vi "FPGAcode5_Debug.vi"(6 "Limits":T1={"High Charge Limit"=4.54747350780585e-13, "Low Charge Limit"=0.0, "High Velocity Limit"=262143.0, "Low Velocity Limit"=0.0, "High Mass Limit"=7.27595761248936e-12, "Low Mass Limit"=0.0, "High Voltage"=2200000.0}, 7 "Speed Bracket":i32, 8 "Thresholds in":i32[](array[numeric])=[0, 0, 0, 0, 0, 0, 0, 0, 0, 0, 0], 9 "Clock Speed (Hz)":i32=40000000, 10 "Calibrate":bool=TRUE, 11 "Detector Waveform In":sgl[][](array[numeric])) -> (0 "Thresholds out":i32[](array[numeric]), 1 "V-M-C Estimate":sgl[](array[numeric]), 3 "PSU Response":bool[](array[boolean]), 5 "Max Stop Point":cluster{"Max Stop":u8, "Index":i32})   [LabVIEW 2015]
uses:
  FPGA3/Detector_Cluster.ctl
  FPGA3/Correlations.ctl
  FPGA3/Limits_In.ctl
panel:
  in  "User Trigger?":bool
  in  "User Trigger Distance":fxp<+/-,34,18> format="%.3g"
  out "User Trigger":bool
  in  "Charge Error Factor":fxp<+,32,0>=0.30000000004656613 format="%_2g"
  in  "Threshold Factor":fxp<+/-,32,16>=1.1999664306640625 format="%.2g"
  out "DCS 2":bool
  out "DCS 1":bool
  in  "Armed":bool
  out "Plates":bool
  in  "One Shot":bool
  # "These factors above are in the front\npanel so it is possible to experiment\nwith different configurations of the\nFPGA on the fly."
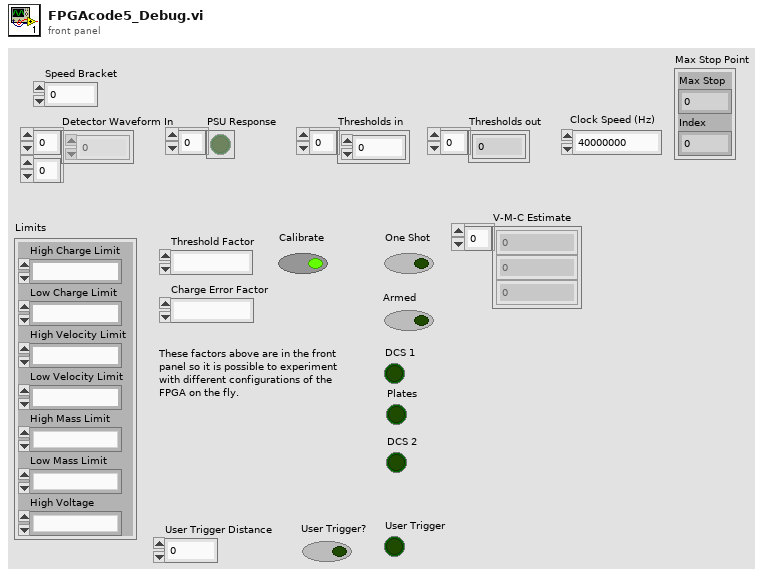
[diagram p1: front panel]
types:
  T1 = typedef "Limits_In.ctl" = cluster{"High Charge Limit":fxp<+,32,-41>, "Low Charge Limit":fxp<+,32,-41>, "High Velocity Limit":fxp<+,18,18>, "Low Velocity Limit":fxp<+,18,18>, "High Mass Limit":fxp<+/-,33,-36>, "Low Mass Limit":fxp<+/-,33,-36>, "High Voltage":fxp<+,32,22>}
  T2 = typedef "Detector_Cluster.ctl" = cluster{"Det 1":i32, "Det 2":i32}
  T3 = cluster{"Filter 1":T2, "Filter 2":T2, "Filter 3":T2, "Filter 4":T2}
  T4 = cluster{"Distance to PSU":fxp<+/-,32,5>, "Distance to end of PSU":fxp<+/-,32,5>, "Distance to DCS 2":fxp<+/-,32,5>, "Distance to DCS 1":fxp<+/-,32,5>, "Distance to front of LEIL Chamber":fxp<+/-,32,5>}
  T5 = cluster{"Detector Max Speed Count":i32, "Detector Min Speed Count":i32, "Gap Max Speed Count":i32, "Gap Min Speed Count":i32}
  T6 = cluster{"Distance to PSU":fxp<+/-,64,37>, "Distance to end of PSU":fxp<+/-,64,37>, "Distance to DCS 2":fxp<+/-,64,37>, "Distance to DCS 1":fxp<+/-,64,37>, "Distance to front of LEIL Chamber":fxp<+/-,64,37>}
  T7 = cluster{"Filter 1":T2, "Filter 2":T2, "Filter 3":T2, "Filter 4":T2}[]
  T8 = cluster{"First Detector Count":i32, "Detector Gap Count":i32, "Second Detector Count":i32, "Second Detector Final Count":i32}
  T9 = typedef "Correlations.ctl" = cluster{"First Correlation":i32, "Latest Correlation":i32}
  T10 = cluster{cluster{i16, i16}, cluster{"Det 1":i16, "Det 2":i16}, cluster{"Det 1":i16, "Det 2":i16}, cluster{"Det 1":i16, "Det 2":i16}}
  T11 = cluster{cluster{"Det 1":i16, "Det 2":i16}, cluster{"Det 1":i16, "Det 2":i16}, cluster{"Det 1":i16, "Det 2":i16}, cluster{"Det 1":i16, "Det 2":i16}}
  T12 = cluster{"Distance to PSU":fxp<+/-,64,69>, "Distance to end of PSU":fxp<+/-,64,69>, "Distance to DCS 2":fxp<+/-,64,69>, "Distance to DCS 1":fxp<+/-,64,69>, "Distance to front of LEIL Chamber":fxp<+/-,64,69>}
  T13 = cluster{"Distance to PSU":i32, "Distance to end of PSU":i32, "Distance to DCS 2":i32, "Distance to DCS 1":i32, "Distance to front of LEIL Chamber":i32}
  T14 = cluster{fxp<+,64,32>, fxp<+/-,64,-31>, "High Charge Limit":fxp<+,32,-41>}
  T15 = cluster{dbl, fxp<+/-,64,-31>, "High Charge Limit":fxp<+,32,-41>}
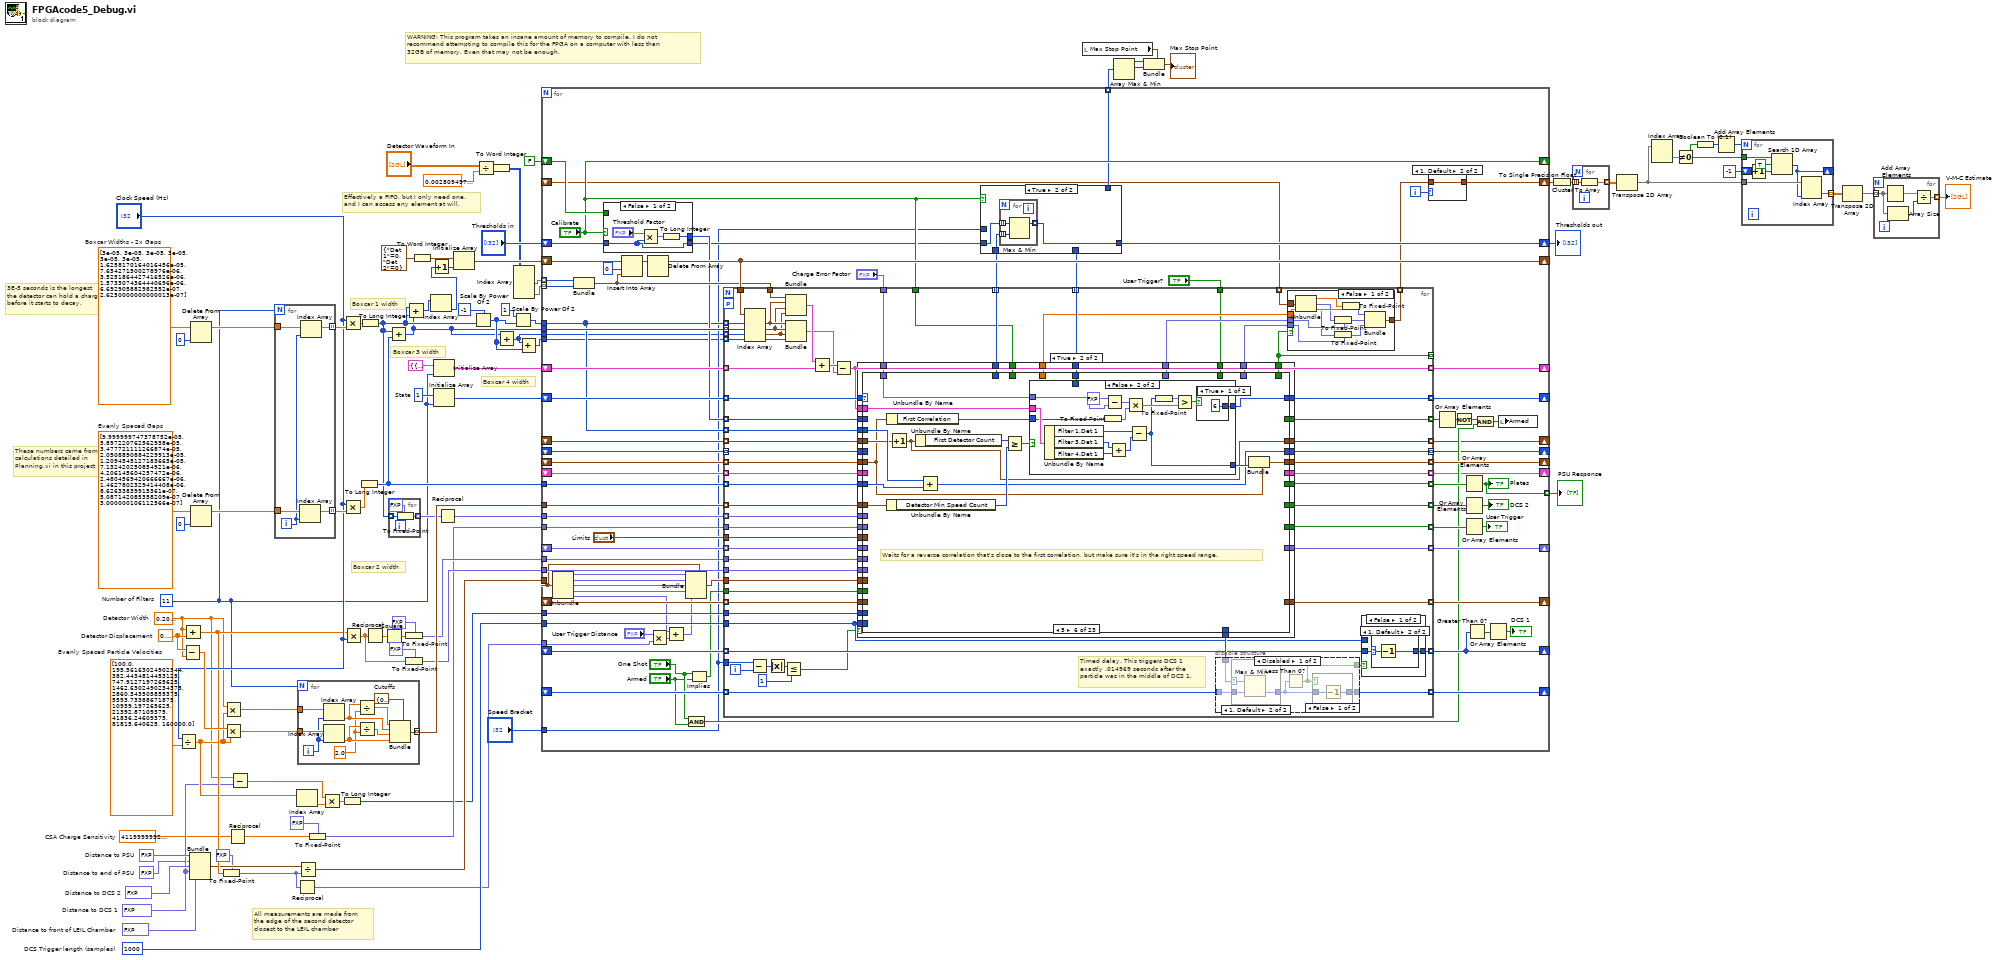
[diagram p0: block diagram]
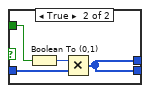
[diagram p3: hidden frame]
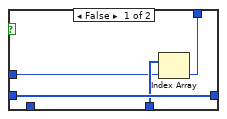
[diagram p4: hidden frame]
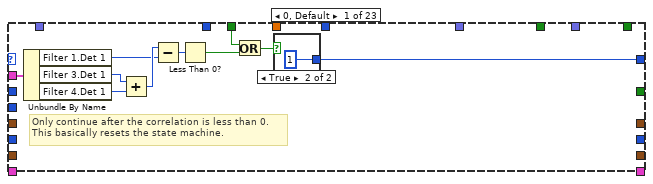
[diagram p6: hidden frame]
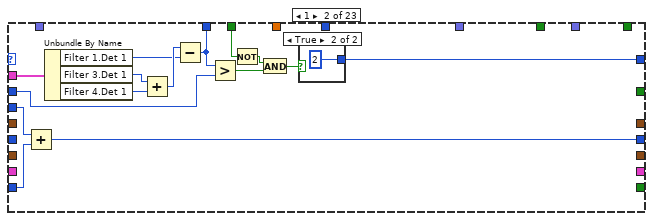
[diagram p8: hidden frame]
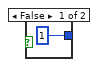
[diagram p9: hidden frame]
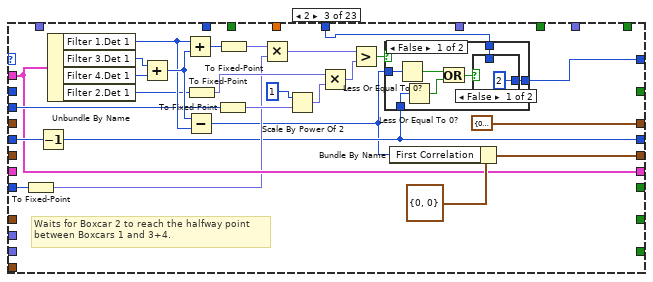
[diagram p10: hidden frame]
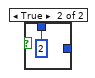
[diagram p11: hidden frame]
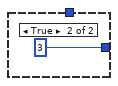
[diagram p12: hidden frame]
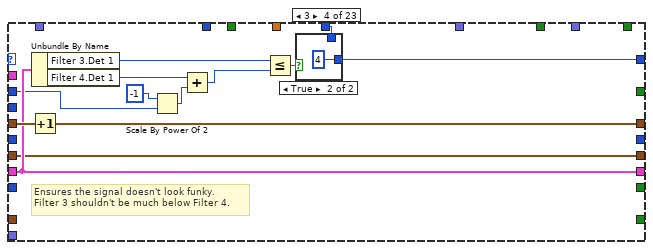
[diagram p13: hidden frame]
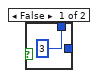
[diagram p14: hidden frame]
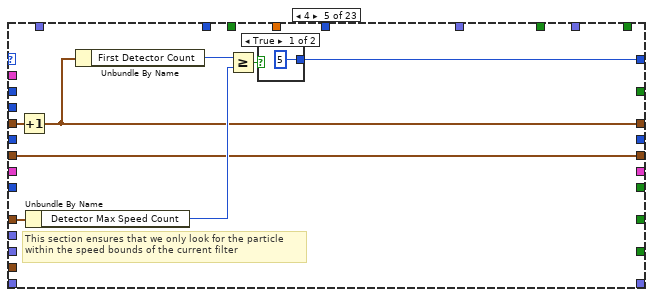
[diagram p15: hidden frame]
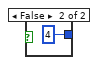
[diagram p16: hidden frame]
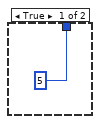
[diagram p17: hidden frame]
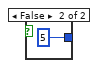
[diagram p18: hidden frame]
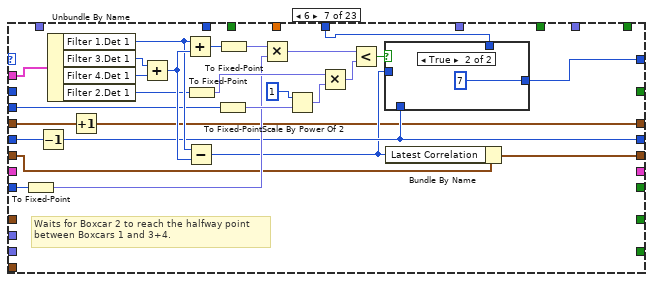
[diagram p19: hidden frame]
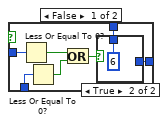
[diagram p20: hidden frame]
diagram:
  w30 = dbl[] [3e-05, 3e-05, 3e-05, 3e-05, 3e-05, 3e-05, 1.6258170164016456e-05, 7.654271500278976e-06, 3.5251864427416526e-06, 1.5733074364440696e-06, 6.692905882982552e-07, 2.6250000000000013e-07]  # Boxcar Widths - 2x Gaps
  w43 = fxp<+/-,32,5> 4.297679997980595  # Distance to front of LEIL Chamber
  w49 = u16 1000  # DCS Trigger length (samples)
  w54 = fxp<+/-,32,5> -1.3589000031352043  # Distance to DCS 1
  w57 = fxp<+/-,32,5> 2.6162000000476837  # Distance to DCS 2
  w46 = fxp<+/-,32,5> 2.7999999970197678  # Distance to end of PSU
  w58 = fxp<+/-,32,5> 0.10000000149011612  # Distance to PSU
  w42 = sgl 4120000000000000.0  # CSA Charge Sensitivity
  w89 = u8 1  # State
  w55 = sgl 0.6  # Detector Displacement
  w93 = sgl[] [0.0001, 5.8972208e-05, 3.477721e-05, 2.050889e-05, 1.2094545e-05, 7.1324203e-06, 4.2061456e-06, 2.480457e-06, 1.4627802e-06, 8.6263384e-07, 5.087142e-07, 3e-07]  # Evenly Spaced Gaps
  w74 = sgl[] [100.0, 195.56163, 382.44348, 747.9127, 1462.6302, 2860.3435, 5593.734, 10939.197, 21392.871, 41836.246, 81815.64, 160000.0]  # Evenly Spaced Particle Velocities
  w50 = sgl 0.21  # Detector Width
  w47 = 11  # Number of Filters
  # "WARNING: This program takes an insane amount of memory to compile. I do not\nrecommend attempting to compile this for the FPGA on a computer with less than\n32GB of memory. Even that may not be enough."
  # "Boxcar 3 width"
  # "Boxcar 4 width"
  # "All measurements are made from\nthe edge of the second detector\nclosest to the LEIL chamber"
  # "Effectively a FIFO, but I only need one,\nand I can access any element at will."
  # "Boxcar 2 width"
  # "Boxcar 1 width"
  # "3E-5 seconds is the longest\nthe detector can hold a charge\nbefore it starts to decay."
  # "These numbers came from\ncalculations detailed in\nPlanning.vi in this project"
  n1 = Divide(x="Clock Speed (Hz)", y=w74) -> (x/y=w56:sgl[])
  n2 = Subtract(x=w55, y=w50) -> (x-y=w73:sgl)
  n3 = Add(x=w50, y=w55) -> (x+y=w61:sgl)
  n4 = Bundle("Distance to PSU"=w58, "Distance to end of PSU"=w46, "Distance to DCS 2"=w57, "Distance to DCS 1"=w54, "Distance to front of LEIL Chamber"=w43) -> (w60:T4)  [unwired: 1 in]
  n5 = Delete From Array(array=w30, index=0) -> (array with subset deleted=w82:dbl[])  [unwired: 1 in, 1 out]
  n6 = Delete From Array(array=w93, index=0) -> (array with subset deleted=w84:sgl[])  [unwired: 1 in, 1 out]
  n7 = To Fixed-Point(fixed-point type=fxp<+/-,32,1> 0.0, number=w61) -> (fixed-point=w45:fxp<+/-,32,1>)
  n8 = Multiply(x=w50, y=w56) -> (x*y=w91:sgl[])
  n9 = Multiply(x=w73, y=w56) -> (x*y=w92:sgl[])
  n10 = Reciprocal(x=w42) -> (1/x=w63:sgl)
  n11 = Subtract(x=w50, y=w54) -> (x-y=w52:sgl)
  n12 = for {
    N: w47 -> [_]
    tunnel: w84 -> [w101]
    tunnel: [w98] -> w83 mode=indexing
    tunnel: w82 -> [w100]
    tunnel: [w99] -> w81 mode=indexing
    i -> [w97]
    n13 = Index Array(array=w101, index=w97) -> (element=w98:sgl)
    n14 = Index Array(array=w100, index=w97) -> (element=w99:dbl)
  }
  n15 = Index Array(array=w56) -> (element=w53:sgl)  [unwired: 1 in]
  n16 = Reciprocal(x=w45) -> (1/x=w44:fxp<+/-,34,33>)
  n17 = for {
    N: w47 -> [_]
    tunnel: w92 -> [w111]
    tunnel: w91 -> [w110]
    tunnel: [w109] -> w86 mode=indexing
    i -> [w108]
    w102 = sgl 2.0 ("y")
    w107 = T5 {"Detector Max Speed Count"=0, "Detector Min Speed Count"=0, "Gap Max Speed Count"=0, "Gap Min Speed Count"=0}  # Cutoffs
    n18 = Index Array(array=w110, index=w108) -> (element=w106:sgl)
    n19 = Index Array(array=w111, index=w108) -> (element=w103:sgl)
    n20 = Divide(x=w106, y=w102) -> (x/y=w105:sgl)
    n21 = Divide(x=w103, y=w102) -> (x/y=w104:sgl)
    n22 = Bundle(cluster=w107, "Detector Max Speed Count"=w105, "Detector Min Speed Count"=w106, "Gap Max Speed Count"=w104, "Gap Min Speed Count"=w103) -> (w109:T5)
  }
  n23 = Divide(x=w60, y=w45) -> (x/y=w59:T6)
  n24 = To Fixed-Point(fixed-point type=fxp<+,32,-49> 0.0, number=w63) -> (fixed-point=w62:fxp<+,32,-49>)
  n25 = Multiply(x=w52, y=w53) -> (x*y=w51:sgl)
  n26 = To Long Integer(number=w51) -> (32bit integer=w48:i32)
  n27 = Multiply(x="Clock Speed (Hz)", y=w81) -> (x*y=w85:dbl[])
  n28 = Multiply(x="Clock Speed (Hz)", y=w83) -> (x*y=w90:sgl[])
  n29 = Multiply(x=w61, y="Clock Speed (Hz)") -> (x*y=w66:sgl)
  n30 = To Long Integer(number=w90) -> (32bit integer=w80:i32[])
  n31 = To Long Integer(number=w85) -> (32bit integer=w6:i32[])
  n32 = Reciprocal(x=w66) -> (1/x=w70:sgl)
  n33 = Square(x=w70) -> (x^2=w69:sgl)
  n34 = Add(x=w6, y=w80) -> (x+y=w2:i32[])
  n35 = for {
    tunnel: w6 -> [w114] mode=indexing
    tunnel: [w113] -> w76 mode=indexing
    n36 = To Fixed-Point(fixed-point type=fxp<+/-,32,32> 0.0, number=w114) -> (fixed-point=w113:fxp<+/-,32,32>)
  }
  n37 = To Fixed-Point(fixed-point type=fxp<+/-,32,-42> 0.0, number=w69) -> (fixed-point=w72:fxp<+/-,32,-42>)
  n38 = To Fixed-Point(fixed-point type=fxp<+,32,28> 0.0, number=w66) -> (fixed-point=w64:fxp<+,32,28>)
  n39 = Add(x=w6, y=w2) -> (x+y=w38:i32[])
  n40 = To Word Integer(number=T2 {"Det 1"=0, "Det 2"=0} ("Detectors")) -> (16bit integer=w79:cluster{"Det 1":i16, "Det 2":i16})
  n41 = Index Array(array=w38) -> (element=w37:i32)  [unwired: 1 in]
  n42 = Increment(x=w37) -> (x+1=w36:i32)
  n43 = Initialize Array(T3 {"Filter 1"={"Det 1"=0, "Det 2"=0}, "Filter 2"={"Det 1"=0, "Det 2"=0}, "Filter 3"={"Det 1"=0, "Det 2"=0}, "Filter 4"={"Det 1"=0, "Det 2"=0}} ("cluster"), w47) -> (w87:T7)
  n44 = Initialize Array(w89, w47) -> (w88:u8[])
  n45 = Reciprocal(x=w76) -> (1/x=w75:fxp<+/-,34,2>[])
  n46 = Initialize Array(w79, w36) -> (w96:cluster{"Det 1":i16, "Det 2":i16}[])
  n47 = Scale By Power Of 2(n=i16 -1, x=w6) -> (x*2^n=w4:i32[])
  n48 = Divide(x="Detector Waveform In", y=sgl 0.0028094975 ("min value")) -> (x/y=w41:sgl[][])
  n49 = To Word Integer(number=w41) -> (16bit integer=w31:i16[][])
  n50 = Add(x=w2, y=w4) -> (x+y=w5:i32[])
  n51 = Scale By Power Of 2(n=i16 1, x=w4) -> (x*2^n=w9:i32[])
  n52 = Index Array(array=w31) -> (element #1=w33:i16[], element #2=w32:i16[])  [unwired: 4 in]
  n53 = Add(x=w5, y=w4) -> (x+y=w3:i32[])
  n54 = for {
    shift-right: [w196] -> _
    shift-left: w96 -> [w197]
    shift-right: [w121] -> _
    shift-left: w87 -> [w193]
    shift-right: [w123] -> _
    shift-left: w88 -> [w195]
    shift-right: [w122] -> _
    shift-left: _ -> [w194]
    tunnel: w86 -> [w192]
    shift-right: [w191] -> _
    shift-left: _ -> [w190]
    tunnel: w9 -> [w120]
    tunnel: w2 -> [w189]
    tunnel: w80 -> [w188]
    tunnel: w75 -> [w187]
    shift-right: [w186] -> _
    shift-left: _ -> [w185]
    tunnel: w72 -> [w184]
    tunnel: w62 -> [w183]
    tunnel: w64 -> [w182]
    tunnel: w59 -> [w169]
    shift-right: [w181] -> _
    shift-left: _ -> [w180]
    shift-right: [w179] -> w39
    shift-left: "Thresholds in" -> [w178]
    shift-right: ["Calibrate"] -> _
    shift-left: FALSE ("Calibrate") -> [w177]
    tunnel: w49 -> [w176]
    tunnel: w48 -> [w175]
    shift-right: [w173] -> _
    shift-left: _ -> [w174]
    shift-right: [w172] -> _
    shift-left: _ -> [w171]
    tunnel: w44 -> [w170]
    tunnel: [w136] -> w29 mode=indexing
    shift-right: [w135] -> _
    shift-left: _ -> [w134]
    tunnel: w33 -> [w133] mode=indexing
    tunnel: w32 -> [w132] mode=indexing
    tunnel: [w128] -> w28 mode=indexing
    tunnel: "Speed Bracket" -> [w117]
    shift-right: [w125] -> w18
    shift-left: _ -> [w127]
    shift-right: [w119] -> _
    shift-left: _ -> [w118]
    tunnel: w3 -> [w116]
    tunnel: w5 -> [w115]
    i -> [w126]
    n55 = Unbundle(w169) -> ("Distance to PSU"=w158:fxp<+/-,64,37>, "Distance to end of PSU"=w157:fxp<+/-,64,37>, "Distance to DCS 2"=w156:fxp<+/-,64,37>, "Distance to DCS 1"=w153:fxp<+/-,64,37>, "Distance to front of LEIL Chamber"=w152:fxp<+/-,64,37>)
    n56 = Bundle(w133, w132) -> (w137:cluster{i16, i16})  [unwired: 1 in]
    n57 = case shown="False" "Calibrate" {
      tunnel: w178 -> [w200 w206]
      tunnel: [w200 w203] -> w129
      tunnel: w177 -> [_ w205]
      tunnel: [w199 w203] -> w130
      frame False {
        n58 = Multiply(x="Threshold Factor", y=w200) -> (x*y=w201:fxp<+/-,64,48>[])
        n59 = To Long Integer(number=w201) -> (32bit integer=w199:i32[])
      }
      frame True {
        n60 = Boolean To (0,1)(Boolean=w205) -> (0, 1=w204:i16)
        n61 = Multiply(x=w204, y=w206) -> (x*y=w203:i32[])
      }
    }
    n62 = Insert Into Array(array=w197, index=0, new element=w137) -> (w168:cluster{"Det 1":i16, "Det 2":i16}[])
    n63 = Delete From Array(array=w168) -> (array with subset deleted=w196:cluster{"Det 1":i16, "Det 2":i16}[])  [unwired: 2 in, 1 out]
    n64 = Multiply(x="User Trigger Distance", y=w170) -> (x*y=w154:fxp<+/-,64,49>)
    n65 = Add(x=w152, y=w154) -> (x+y=w151:fxp<+/-,64,50>)
    n66 = Bundle(cluster=w169, "Distance to PSU"=w158, "Distance to end of PSU"=w157, "Distance to DCS 2"=w156, "Distance to DCS 1"=w153, "Distance to front of LEIL Chamber"=w151) -> (w155:T6)
    n67 = And(x="One Shot", y="Armed") -> (x .and. y?=w142:bool)
    n68 = Implies(1:"Armed", 2:"One Shot") -> (0:w162:bool)
    n69 = for {
      tunnel: w196 -> [w285]
      tunnel: [w271] -> w121 mode=indexing
      tunnel: w195 -> [w284] mode=indexing
      tunnel: [w283] -> w123 mode=indexing
      tunnel: w130 -> [w220] mode=indexing
      tunnel: [w282] -> w122 mode=indexing
      tunnel: w194 -> [w281] mode=indexing
      tunnel: w193 -> [w275] mode=indexing
      tunnel: w137 -> [w280]
      tunnel: w192 -> [w270] mode=indexing
      tunnel: [w269] -> w191 mode=indexing
      tunnel: w190 -> [w268] mode=indexing
      tunnel: w120 -> [w267] mode=indexing
      tunnel: w189 -> [w218] mode=indexing
      tunnel: w115 -> [w266] mode=indexing
      tunnel: w116 -> [w265] mode=indexing
      tunnel: w120 -> [w226] mode=indexing
      tunnel: w188 -> [w225] mode=indexing
      tunnel: "Charge Error Factor" -> [w264]
      tunnel: [w263] -> w164 mode=indexing
      tunnel: w187 -> [w262] mode=indexing
      tunnel: "Limits" -> [w261]
      tunnel: [w260] -> w186 mode=indexing
      tunnel: w185 -> [w259] mode=indexing
      tunnel: w184 -> [w258]
      tunnel: w183 -> [w257]
      tunnel: w182 -> [w256]
      tunnel: w155 -> [w255]
      tunnel: [w254] -> w181 mode=indexing
      tunnel: w180 -> [w253] mode=indexing
      tunnel: [w252] -> w163 mode=indexing
      tunnel: w162 -> [w251]
      tunnel: w176 -> [w248]
      tunnel: w175 -> [w250]
      tunnel: [w247] -> w173 mode=indexing
      tunnel: w174 -> [w246] mode=indexing
      tunnel: [w244] -> w172 mode=indexing
      tunnel: w171 -> [w243] mode=indexing
      tunnel: [w242] -> w150 mode=indexing
      tunnel: [w241] -> w149 mode=indexing
      tunnel: [w240] -> w148 mode=indexing
      tunnel: [w239] -> w145 mode=indexing
      tunnel: "User Trigger?" -> [w235]
      tunnel: w134 -> [w233] mode=indexing
      tunnel: [w232] -> w135 mode=indexing
      tunnel: "Calibrate" -> [w231]
      tunnel: [w224] -> w124 mode=indexing
      tunnel: w127 -> [w230] mode=indexing
      workers-P: _ -> [_]
      tunnel: w117 -> [w221]
      tunnel: [w223] -> _ mode=indexing
      tunnel: [w219] -> w119 mode=indexing
      tunnel: w118 -> [w217] mode=indexing
      i -> [w222]
      # "Timed delay. This triggers DCS 1\nexactly .014969 seconds after the\nparticle was in the middle of DCS 1."
      n70 = Index Array(array=w285, index #1=w267, index #2=w218, index #3=w266, index #4=w265) -> (element #1=w278:cluster{"Det 1":i16, "Det 2":i16}, element #2=w277:cluster{"Det 1":i16, "Det 2":i16}, element #3=w276:cluster{"Det 1":i16, "Det 2":i16}, element #4=w279:cluster{"Det 1":i16, "Det 2":i16})
      n71 = Subtract(x=w221, y=w222) -> (x-y=w234:i32)
      n72 = Absolute Value(x=w234) -> (abs(x)=w229:i32)
      n73 = Less Or Equal?(x=w229, y=1) -> (x <= y?=w228:bool)
      n74 = Bundle(w280, w278, w277, w276) -> (w274:T10)  [unwired: 1 in]
      n75 = Bundle(w278, w277, w276, w279) -> (w272:T11)  [unwired: 1 in]
      n76 = Add(x=w274, y=w275) -> (x+y=w273:T3)
      n77 = Subtract(x=w273, y=w272) -> (x-y=w271:T3)
      n78 = case shown="True" w228 {
        tunnel: w284 -> [_ w327]
        tunnel: w220 -> [_ w326]
        tunnel: [_ w325] -> w283
        tunnel: [_ w324] -> w282
        tunnel: w281 -> [_ w323]
        tunnel: w217 -> [_ w322]
        tunnel: w271 -> [_ w321]
        tunnel: w270 -> [_ w320]
        tunnel: [_ w319] -> w269
        tunnel: w268 -> [_ w318]
        tunnel: w225 -> [_ w317]
        tunnel: w264 -> [_ w316]
        tunnel: [_ w315] -> w263
        tunnel: w262 -> [_ w314]
        tunnel: w261 -> [_ w313]
        tunnel: [_ w312] -> w260
        tunnel: w259 -> [_ w311]
        tunnel: w258 -> [_ w310]
        tunnel: w257 -> [_ w309]
        tunnel: w256 -> [_ w308]
        tunnel: w255 -> [_ w307]
        tunnel: [_ w306] -> w254
        tunnel: w253 -> [_ w305]
        tunnel: [_ w304] -> w252
        tunnel: w251 -> [_ w303]
        tunnel: w250 -> [_ w302]
        tunnel: [_ w301] -> w249
        tunnel: w248 -> [_ w300]
        tunnel: [_ w299] -> w242
        tunnel: [_ w298] -> w241
        tunnel: [_ w297] -> w240
        tunnel: [_ w296] -> w239
        tunnel: [_ w295] -> w238
        tunnel: [_ w294] -> w237
        tunnel: [_ w293] -> w236
        tunnel: w226 -> [_ w292]
        tunnel: w235 -> [_ w291]
        tunnel: [_ w290] -> w232
        tunnel: w233 -> [_ w289]
        tunnel: [_ w288] -> w223
        tunnel: w231 -> [_ w287]
        tunnel: [_ w286] -> w219
        frame False {
        }
        frame True {
          n79 = case shown="5" w327 {
            tunnel: w326 -> [_ w353 _ w393 _ _ _ _ _ _ _ _ _ _ _ _ _ _ _ _ _ _ _]
            tunnel: [w336 w351 w380 w404 w410 w425 w477 w510 w554 w567 w583 w638 w668 w687 w739 w790 u8 17 ("Det 3") w823 w831 w838 w852 w858 w871] -> w325
            tunnel: w292 -> [_ w341 w371 _ _ w427 w469 _ _ _ w585 _ _ w689 _ _ w814 _ _ _ _ _ _]
            tunnel: [_ _ T8 {"First Detector Count"=0, "Detector Gap Count"=0, "Second Detector Count"=0, "Second Detector Final Count"=0} ("Cutoffs") w398 w407 w417 w452 w508 w550 w572 _ w636 w673 _ w737 _ _ _ _ _ _ _ _] -> w324
            tunnel: w323 -> [_ _ _ w403 w408 w422 w453 w507 w549 w572 w582 w635 w673 w686 w736 _ _ _ _ _ _ _ _]
            tunnel: w322 -> [_ _ w381 _ _ _ w478 w513 _ _ _ w641 _ _ w742 _ _ _ _ _ _ _ _]
            tunnel: w321 -> [w331 w346 w364 _ _ w428 w462 w489 _ _ w586 w633 _ w682 w734 _ _ _ _ _ _ _ _]
            tunnel: w320 -> [_ _ _ _ w414 w433 _ w499 _ w571 w591 w626 w672 w693 w727 _ _ _ _ _ _ _ _]
            tunnel: [_ _ w366 w399 w409 w421 w464 w503 w552 w570 w579 w630 w671 w680 w731 w802 _ _ _ _ _ _ _] -> w319
            tunnel: w318 -> [_ _ _ w399 w409 w419 w454 w511 w553 w573 w592 w639 w674 w694 w740 w803 w821 _ _ _ _ _ _]
            tunnel: w317 -> [_ w340 w372 _ _ w426 w470 _ _ _ w584 _ _ w688 _ _ _ _ _ _ _ _ _]
            tunnel: w316 -> [_ _ _ _ _ w429 _ w491 _ _ w587 w618 _ w690 w721 _ _ _ _ _ _ _ _]
            tunnel: [_ _ w357 w402 _ w430 w456 w493 w555 _ w588 w620 _ w691 w723 w789 _ _ _ _ _ _ _] -> w315
            tunnel: w314 -> [_ _ _ _ _ _ _ _ w560 _ _ _ _ _ _ _ _ _ _ _ _ _ _]
            tunnel: w313 -> [_ _ _ _ _ _ _ _ w563 _ _ _ _ _ _ w804 _ _ _ _ _ _ _]
            tunnel: [_ _ _ _ _ _ _ _ w538 w566 w576 w616 w667 w684 w719 _ _ _ _ _ _ _ _] -> w312
            tunnel: w311 -> [_ _ _ _ _ _ _ _ _ w566 w576 w616 w667 w684 w719 w776 _ _ _ _ _ _ _]
            tunnel: w310 -> [_ _ _ _ _ _ _ _ _ _ _ _ _ _ _ w800 _ _ _ _ _ _ _]
            tunnel: w309 -> [_ _ _ _ _ _ _ _ w547 _ _ _ _ _ _ _ _ _ _ _ _ _ _]
            tunnel: w308 -> [_ _ _ _ _ _ _ _ _ _ _ _ _ _ _ w774 _ _ _ _ _ _ _]
            tunnel: w307 -> [_ _ _ _ _ _ _ _ _ _ _ _ _ _ _ _ w818 _ _ _ _ _ _]
            tunnel: [_ _ _ _ _ _ _ _ _ _ _ _ _ _ _ _ w811 w825 w833 w840 w849 w860 w869] -> w306
            tunnel: w305 -> [_ _ _ _ _ _ _ _ _ _ _ _ _ _ _ _ _ w826 w834 w841 w850 w861 w870]
            tunnel: [_ w345 _ _ _ _ _ _ _ _ _ _ _ _ _ _ _ _ _ _ _ _ _] -> w304
            tunnel: w303 -> [_ _ _ _ _ _ _ _ _ _ _ _ _ _ _ w783 _ _ _ _ _ _ _]
            tunnel: w302 -> [_ _ _ _ _ _ _ _ _ _ _ _ _ _ _ _ w810 _ _ _ _ _ _]
            tunnel: w300 -> [_ _ _ _ _ _ _ _ _ _ _ _ _ _ _ _ _ _ _ _ w847 _ w867]
            tunnel: [_ _ _ _ _ _ _ _ _ _ _ _ _ _ _ _ w808 _ _ _ _ _ _] -> w301
            tunnel: [_ _ _ _ _ _ _ _ _ _ _ _ _ _ _ _ _ _ TRUE _ _ _ _] -> w299
            tunnel: [_ _ _ _ _ _ _ _ _ _ _ _ _ _ _ _ _ _ _ _ TRUE _ _] -> w298
            tunnel: [_ _ _ _ _ _ _ _ _ _ _ _ _ _ _ _ _ _ _ _ _ _ TRUE] -> w297
            tunnel: [_ _ _ _ _ _ _ _ _ _ _ _ _ _ _ w782 _ _ _ _ _ _ _] -> w296
            tunnel: [_ _ _ _ _ _ _ _ _ _ _ _ _ _ _ w773 _ _ _ _ _ _ _] -> w293
            tunnel: [_ _ _ _ _ _ _ _ w538 _ _ _ _ _ _ w776 _ _ _ _ _ _ _] -> w295
            tunnel: [_ _ _ _ _ _ _ _ _ _ _ _ _ _ _ w771 _ _ _ _ _ _ _] -> w294
            tunnel: w291 -> [_ _ _ _ _ _ _ _ _ _ _ _ _ _ _ _ _ _ _ _ w844 _ _]
            tunnel: [_ _ w364 w400 _ _ _ _ _ _ _ _ _ _ _ _ _ _ _ _ _ _ _] -> w290
            tunnel: w289 -> [_ _ _ w400 _ _ _ _ _ _ _ _ _ _ _ _ _ _ _ _ _ _ _]
            tunnel: [_ _ _ _ _ _ _ _ TRUE ("result") _ _ _ _ _ _ TRUE ("result") _ _ _ _ _ _ _] -> w288
            tunnel: w287 -> [w328 w342 _ _ _ _ _ _ _ _ _ _ _ _ _ _ _ _ _ _ _ _ _]
            tunnel: [_ w339 w360 _ _ w418 w458 _ _ _ _ _ _ _ _ _ _ _ _ _ _ _ _] -> w286
            frame 0, Default {
              # "Only continue after the correlation is less than 0.\nThis basically resets the state machine."
              n80 = Unbundle By Name(w331) -> ("Filter 1.Det 1"=w332:i32, "Filter 3.Det 1"=w333:i32, "Filter 4.Det 1"=w334:i32)
              n81 = Add(x=w333, y=w334) -> (x+y=w335:i32)
              n82 = Subtract(x=w335, y=w332) -> (x-y=w330:i32)
              n83 = Less Than 0?(x=w330) -> (x < 0?=w337:bool)
              n84 = Or(x=w328, y=w337) -> (x .or. y?=w329:bool)
              n85 = case shown="True" w329 {
                tunnel: [_ u8 1 ("Det 3")] -> w336
                frame False {
                }
                frame True {
                }
              }
            }
            frame 1 {
              n86 = Add(x=w341, y=w340) -> (x+y=w339:i32)
              n87 = Unbundle By Name(w346) -> ("Filter 1.Det 1"=w347:i32, "Filter 3.Det 1"=w348:i32, "Filter 4.Det 1"=w349:i32)
              n88 = Add(x=w348, y=w349) -> (x+y=w350:i32)
              n89 = Subtract(x=w350, y=w347) -> (x-y=w345:i32)
              n90 = Greater?(x=w345, y=w353) -> (0:w352:bool)
              n91 = Not(x=w342) -> (.not. x?=w343:bool)
              n92 = And(x=w343, y=w352) -> (x .and. y?=w344:bool)
              n93 = case shown="True" w344 {
                tunnel: [u8 1 ("Det 3") u8 2 ("Det 3")] -> w351
                frame False {
                }
                frame True {
                }
              }
            }
            frame 2 {
              # "Waits for Boxcar 2 to reach the halfway point\nbetween Boxcars 1 and 3+4."
              n94 = To Fixed-Point(number=w372) -> (fixed-point=w361:fxp<+/-,32,32>)  [unwired: 1 in]
              n95 = Decrement(x=w381) -> (x-1=w360:i32)
              n96 = Unbundle By Name(w364) -> ("Filter 1.Det 1"=w374:i32, "Filter 3.Det 1"=w378:i32, "Filter 4.Det 1"=w377:i32, "Filter 2.Det 1"=w368:i32)
              n97 = Add(x=w378, y=w377) -> (x+y=w375:i32)
              n98 = Add(x=w374, y=w375) -> (x+y=w379:i32)
              n99 = Subtract(x=w375, y=w374) -> (x-y=w356:i32)
              n100 = To Fixed-Point(number=w368) -> (fixed-point=w363:fxp<+/-,32,32>)  [unwired: 1 in]
              n101 = To Fixed-Point(number=w371) -> (fixed-point=w362:fxp<+/-,32,32>)  [unwired: 1 in]
              n102 = To Fixed-Point(number=w379) -> (fixed-point=w365:fxp<+/-,32,32>)  [unwired: 1 in]
              n103 = Multiply(x=w365, y=w361) -> (x*y=w373:fxp<+/-,64,64>)
              n104 = Scale By Power Of 2(n=i16 1, x=w362) -> (x*2^n=w369:fxp<+/-,32,32>)
              n105 = Multiply(x=w363, y=w369) -> (x*y=w367:fxp<+/-,64,64>)
              n106 = Greater?(x=w373, y=w367) -> (0:w358:bool)
              n107 = case shown="False" w358 {
                tunnel: [w388 u8 3 ("Det 3")] -> w380
                tunnel: w360 -> [w383 _]
                tunnel: [w387 _] -> w357
                tunnel: w356 -> [w382 _]
                frame False {
                  n108 = Less Or Equal To 0?(x=w382) -> (x <= 0?=w385:bool)
                  n109 = Less Or Equal To 0?(x=w383) -> (x <= 0?=w384:bool)
                  n110 = Or(x=w385, y=w384) -> (x .or. y?=w386:bool)
                  n111 = case shown="False" w386 {
                    tunnel: [u8 2 ("Det 3") _] -> w388
                    tunnel: [_ u8 2 ("Det 3")] -> w387
                    frame False {
                    }
                    frame True {
                    }
                  }
                }
                frame True {
                }
              }
              n112 = Bundle By Name(cluster=T9 {"First Correlation"=0, "Latest Correlation"=0}, "First Correlation"=w356) -> (w366:T9)
            }
            frame 3 {
              # "Ensures the signal doesn't look funky.\nFilter 3 shouldn't be much below Filter 4."
              n113 = Increment(x=w403) -> (x+1=w398:T8)
              n114 = Unbundle By Name(w400) -> ("Filter 3.Det 1"=w397:i32, "Filter 4.Det 1"=w396:i32)
              n115 = Scale By Power Of 2(n=i16 -1, x=w393) -> (x*2^n=w392:i32)
              n116 = Add(x=w396, y=w392) -> (x+y=w395:i32)
              n117 = Less Or Equal?(x=w397, y=w395) -> (x <= y?=w401:bool)
              n118 = case shown="True" w401 {
                tunnel: [_ u8 4] -> w404
                tunnel: [u8 3 _] -> w402
                frame False {
                }
                frame True {
                }
              }
            }
            frame 4 {
              # "This section ensures that we only look for the particle\nwithin the speed bounds of the current filter"
              n119 = Increment(x=w408) -> (x+1=w407:T8)
              n120 = Unbundle By Name(w414) -> ("Detector Max Speed Count"=w412:i32)
              n121 = Unbundle By Name(w407) -> ("First Detector Count"=w413:i32)
              n122 = Greater Or Equal?(x=w413, y=w412) -> (x >= y?=w411:bool)
              n123 = case shown="True" w411 {
                tunnel: [u8 5 u8 4] -> w410
                frame True {
                }
                frame False {
                }
              }
            }
            frame 5 {
              # "Waits for a reverse correlation that's close to the first correlation, but make sure it's in the right speed range."
              n124 = Unbundle By Name(w433) -> ("Detector Min Speed Count"=w432:i32)
              n125 = Unbundle By Name(w419) -> ("First Correlation"=w424:i32)
              n126 = Increment(x=w422) -> (x+1=w417:T8)
              n127 = Unbundle By Name(w417) -> ("First Detector Count"=w423:i32)
              n128 = Add(x=w427, y=w426) -> (x+y=w418:i32)
              n129 = Greater Or Equal?(x=w423, y=w432) -> (x >= y?=w431:bool)
              n130 = case shown="False" w431 {
                tunnel: [_ w449] -> w425
                tunnel: [u8 5 _] -> w430
                tunnel: w429 -> [_ w448]
                tunnel: w428 -> [_ w445]
                tunnel: w424 -> [_ w436]
                tunnel: [_ w435] -> w420
                frame True {
                }
                frame False {
                  n131 = Unbundle By Name(w445) -> ("Filter 1.Det 1"=w442:i32, "Filter 3.Det 1"=w444:i32, "Filter 4.Det 1"=w443:i32)
                  n132 = To Fixed-Point(number=w436) -> (fixed-point=w438:fxp<+/-,32,32>)  [unwired: 1 in]
                  n133 = Subtract(x=fxp<+,1,1> 1.0, y=w448) -> (x-y=w446:fxp<+,33,1>)
                  n134 = Add(x=w444, y=w443) -> (x+y=w441:i32)
                  n135 = Multiply(x=w446, y=w438) -> (x*y=w440:fxp<+/-,64,32>)
                  n136 = Subtract(x=w442, y=w441) -> (x-y=w435:i32)
                  n137 = To Fixed-Point(number=w435) -> (fixed-point=w437:fxp<+/-,32,32>)  [unwired: 1 in]
                  n138 = Greater?(x=w437, y=w440) -> (0:w439:bool)
                  n139 = case shown="True" w439 {
                    tunnel: [u8 6 u8 5] -> w449
                    frame True {
                    }
                    frame False {
                    }
                  }
                }
              }
              n140 = Bundle(cluster=w419, "Latest Correlation"=w420) -> (w421:T9)  [unwired: 1 in]
            }
            frame 6 {
              # "Waits for Boxcar 2 to reach the halfway point\nbetween Boxcars 1 and 3+4."
              n141 = To Fixed-Point(number=w470) -> (fixed-point=w459:fxp<+/-,32,32>)  [unwired: 1 in]
              n142 = Decrement(x=w478) -> (x-1=w458:i32)
              n143 = Unbundle By Name(w462) -> ("Filter 1.Det 1"=w472:i32, "Filter 3.Det 1"=w475:i32, "Filter 4.Det 1"=w474:i32, "Filter 2.Det 1"=w466:i32)
              n144 = Increment(x=w453) -> (x+1=w452:T8)
              n145 = Add(x=w475, y=w474) -> (x+y=w473:i32)
              n146 = Add(x=w472, y=w473) -> (x+y=w476:i32)
              n147 = Subtract(x=w472, y=w473) -> (x-y=w455:i32)
              n148 = To Fixed-Point(number=w466) -> (fixed-point=w461:fxp<+/-,32,32>)  [unwired: 1 in]
              n149 = To Fixed-Point(number=w469) -> (fixed-point=w460:fxp<+/-,32,32>)  [unwired: 1 in]
              n150 = To Fixed-Point(number=w476) -> (fixed-point=w463:fxp<+/-,32,32>)  [unwired: 1 in]
              n151 = Multiply(x=w463, y=w459) -> (x*y=w471:fxp<+/-,64,64>)
              n152 = Scale By Power Of 2(n=i16 1, x=w460) -> (x*2^n=w467:fxp<+/-,32,32>)
              n153 = Multiply(x=w461, y=w467) -> (x*y=w465:fxp<+/-,64,64>)
              n154 = Less?(x=w471, y=w465) -> (x < y?=w457:bool)
              n155 = case shown="True" w457 {
                tunnel: [w485 u8 7 ("Det 3")] -> w477
                tunnel: w458 -> [w480 _]
                tunnel: [w484 _] -> w456
                tunnel: w455 -> [w479 _]
                frame False {
                  n156 = Less Or Equal To 0?(x=w479) -> (x <= 0?=w482:bool)
                  n157 = Less Or Equal To 0?(x=w480) -> (x <= 0?=w481:bool)
                  n158 = Or(x=w482, y=w481) -> (x .or. y?=w483:bool)
                  n159 = case shown="True" w483 {
                    tunnel: [u8 6 ("Det 3") _] -> w485
                    tunnel: [_ u8 6 ("Det 3")] -> w484
                    frame False {
                    }
                    frame True {
                    }
                  }
                }
                frame True {
                }
              }
              n160 = Bundle By Name(cluster=w454, "Latest Correlation"=w455) -> (w464:T9)
            }
            frame 7 {
              # "Searches for a maximum correlation. If the maximum correlation happens\nafter the speed limit, this isn't the right filter, and we go back to the beginning.\nIf the maximum correlation is too big, we also go back to the beginning."
              n161 = Decrement(x=w513) -> (x-1=w512:i32)
              n162 = Unbundle By Name(w489) -> ("Filter 1.Det 1"=w495:i32, "Filter 3.Det 1"=w505:i32, "Filter 4.Det 1"=w504:i32)
              n163 = Unbundle By Name(w499) -> ("Detector Min Speed Count"=w497:i32)
              n164 = Unbundle By Name(w507) -> ("Detector Gap Count"=w501:i32)
              n165 = Add(x=w505, y=w504) -> (x+y=w494:i32)
              n166 = Subtract(x=w495, y=w494) -> (x-y=w506:i32)
              n167 = Increment(x=w511) -> (x+1=w500:T9)
              n168 = Add(x=w501) -> (x+y=w502:i32)  [unwired: 1 in]
              n169 = Greater?(x=w506, y=w502) -> (0:w509:bool)
              n170 = case shown="True" w509 {
                tunnel: [w520 w536] -> w503
                tunnel: w500 -> [w520 w533]
                tunnel: w506 -> [_ w527]
                tunnel: [w521 w535] -> w508
                tunnel: w507 -> [w521 w534]
                tunnel: [_ w532] -> w498
                tunnel: w491 -> [_ w531]
                tunnel: [_ w525] -> w490
                frame False {
                }
                frame True {
                  w524 = fxp<+/-,32,32> 0.0 ("fixed-point type")
                  n171 = Unbundle(w533) -> ("First Correlation"=w532:i32)  [unwired: 1 out]
                  n172 = Unbundle(w534) -> ("First Detector Count"=w530:i32)  [unwired: 3 out]
                  n173 = Increment(x=w531) -> (x+1=w522:fxp<+,33,1>)
                  n174 = Bundle(cluster=w533, "First Correlation"=w532, "Latest Correlation"=0 ("Detector Gap Count")) -> (w536:T9)
                  n175 = To Fixed-Point(fixed-point type=w524, number=w530) -> (fixed-point=w529:fxp<+/-,32,32>)
                  n176 = Bundle(cluster=w534, "First Detector Count"=w530, "Detector Gap Count"=w527) -> (w535:T8)  [unwired: 2 in]
                  n177 = To Fixed-Point(fixed-point type=w524, number=w527) -> (fixed-point=w526:fxp<+/-,32,32>)
                  n178 = Multiply(x=w522, y=w529) -> (x*y=w528:fxp<+/-,64,33>)
                  n179 = Less?(x=w528, y=w526) -> (x < y?=w525:bool)
                }
              }
              n180 = Greater?(x=w498, y=w497) -> (0:w496:bool)
              n181 = Or(x=w490, y=w496) -> (x .or. y?=w492:bool)
              n182 = case shown="False" w492 {
                tunnel: w512 -> [w516 _]
                tunnel: [w515 _] -> w510
                tunnel: [_ u8 7 ("Det 3")] -> w493
                frame False {
                  n183 = Less Or Equal To 0?(x=w516) -> (x <= 0?=w514:bool)
                  n184 = case shown="True" w514 {
                    tunnel: [u8 8 ("Det 3") u8 7 ("Det 3")] -> w515
                    frame True {
                    }
                    frame False {
                    }
                  }
                }
                frame True {
                }
              }
            }
            frame 8 {
              # "q = ADC value / CSA sensitivity"
              # "Ensures the charge is good"
              n185 = Unbundle(w549) -> ("First Detector Count"=w562:i32, "Detector Gap Count"=w561:i32)  [unwired: 2 out]
              n186 = Unbundle By Name(w563) -> ("High Charge Limit"=w539:fxp<+,32,-41>, "Low Charge Limit"=w559:fxp<+,32,-41>)
              n187 = Add(x=w562, y=w561) -> (x+y=w542:i32)
              n188 = Scale By Power Of 2(n=i16 -1, x=w542) -> (x*2^n=w540:i32)
              n189 = To Fixed-Point(fixed-point type=fxp<+/-,32,32> 0.0, number=w540) -> (fixed-point=w541:fxp<+/-,32,32>)
              n190 = Multiply(x=w541, y=w560) -> (x*y=w548:fxp<+/-,64,33>)
              n191 = Increment(x=w553) -> (x+1=w552:T9)
              n192 = To Long Integer(number=w540) -> (32bit integer=w551:i32)
              n193 = Multiply(x=w548, y=w547) -> (x*y=w546:fxp<+/-,64,-16>)
              n194 = Bundle(cluster=w549, "First Detector Count"=w551, "Detector Gap Count"=0 ("Latest Correlation")) -> (w550:T8)  [unwired: 2 in]
              n195 = To Fixed-Point(fixed-point type=w539, number=w546) -> (fixed-point=w538:fxp<+,32,-41>)
              n196 = Less?(x=w538, y=w539) -> (x < y?=w558:bool)
              n197 = Greater?(x=w538, y=w559) -> (0:w557:bool)
              n198 = And(x=w558, y=w557) -> (x .and. y?=w556:bool)
              n199 = case shown="True" w556 {
                tunnel: [_ u8 8 ("Det 3")] -> w555
                tunnel: [u8 9 ("Det 3") _] -> w554
                frame True {
                }
                frame False {
                }
              }
            }
            frame 9 {
              # "Wait for the particle to get to the second detector."
              n200 = Increment(x=w573) -> (x+1=w570:T9)
              n201 = Unbundle By Name(w571) -> ("Gap Max Speed Count"=w569:i32)
              n202 = Unbundle By Name(w570) -> ()  [unwired: 1 out]
              n203 = Greater Or Equal?(y=w569) -> (x >= y?=w568:bool)  [unwired: 1 in]
              n204 = case shown="True" w568 {
                tunnel: [u8 10 ("State") u8 9 ("State")] -> w567
                frame True {
                }
                frame False {
                }
              }
            }
            frame 10 {
              (unwired) 0 ("Second Detector Count")
              # "Waits for a correlation that's close to the first two correlations."
              n205 = Increment(x=w592) -> (x+1=w578:T9)
              n206 = Unbundle By Name(w582) -> ("First Detector Count"=w581:i32)
              n207 = Unbundle By Name(w591) -> ("Gap Min Speed Count"=w590:i32)
              n208 = Unbundle(w578) -> ("First Correlation"=w580:i32, "Latest Correlation"=w577:i32)
              n209 = Greater Or Equal?(x=w577, y=w590) -> (x >= y?=w589:bool)
              n210 = case shown="False" w589 {
                tunnel: [_ w613] -> w583
                tunnel: [u8 10 _] -> w588
                tunnel: w587 -> [_ w612]
                tunnel: w586 -> [_ w609]
                tunnel: w581 -> [_ w599]
                tunnel: [_ w597] -> _
                frame True {
                }
                frame False {
                  w596 = fxp<+/-,32,32> 0.0 ("fixed-point type")
                  n211 = Scale By Power Of 2(n=i16 0, x=w612) -> (x*2^n=w595:fxp<+,32,0>)
                  n212 = Unbundle By Name(w609) -> ("Filter 1.Det 2"=w606:i32, "Filter 3.Det 2"=w608:i32, "Filter 4.Det 2"=w607:i32)
                  n213 = To Fixed-Point(fixed-point type=w596, number=w599) -> (fixed-point=w602:fxp<+/-,32,32>)
                  n214 = Subtract(x=fxp<+,1,1> 1.0, y=w595) -> (x-y=w610:fxp<+,33,1>)
                  n215 = Add(x=w608, y=w607) -> (x+y=w605:i32)
                  n216 = Multiply(x=w610, y=w602) -> (x*y=w604:fxp<+/-,64,32>)
                  n217 = Subtract(x=w605, y=w606) -> (x-y=w598:i32)
                  n218 = To Fixed-Point(fixed-point type=w596, number=w598) -> (fixed-point=w601:fxp<+/-,32,32>)
                  n219 = Greater?(x=w601, y=w604) -> (0:w603:bool)
                  n220 = case shown="True" w603 {
                    tunnel: [u8 11 u8 10] -> w613
                    frame True {
                    }
                    frame False {
                    }
                  }
                  n221 = Bundle(cluster=T9 {"First Correlation"=0, "Latest Correlation"=0} ("input cluster"), "First Correlation"=w599, "Latest Correlation"=w598) -> (w597:T9)
                }
              }
              n222 = Add(x=w585, y=w584) -> ()  [unwired: 1 out]
              n223 = Bundle(cluster=w578, "First Correlation"=w580, "Latest Correlation"=w577) -> (w579:T9)
            }
            frame 11 {
              # "Searches for a maximum correlation. If the maximum correlation happens\nafter the speed limit, this isn't the right filter, and we go back to the beginning.\nIf the maximum correlation is too big, we also go back to the beginning."
              n224 = Decrement(x=w641) -> (x-1=w640:i32)
              n225 = Unbundle By Name(w633) -> ("Filter 1.Det 2"=w622:i32, "Filter 3.Det 2"=w632:i32, "Filter 4.Det 2"=w631:i32)
              n226 = Unbundle By Name(w626) -> ("Gap Min Speed Count"=w624:i32)
              n227 = Unbundle By Name(w635) -> ("Detector Gap Count"=w628:i32)
              n228 = Add(x=w632, y=w631) -> (x+y=w621:i32)
              n229 = Subtract(x=w621, y=w622) -> (x-y=w634:i32)
              n230 = Increment(x=w639) -> (x+1=w627:T9)
              n231 = Add(x=w628) -> (x+y=w629:i32)  [unwired: 1 in]
              n232 = Greater?(x=w634, y=w629) -> (0:w637:bool)
              n233 = case shown="True" w637 {
                tunnel: [w648 w666] -> w630
                tunnel: w627 -> [w648 w663]
                tunnel: w634 -> [_ w657]
                tunnel: [w649 w665] -> w636
                tunnel: w635 -> [w649 w664]
                tunnel: [_ w654] -> w625
                tunnel: w618 -> [_ w661]
                tunnel: [_ w655] -> w617
                frame False {
                }
                frame True {
                  (unwired) 0 ("Second Detector Count")
                  w653 = fxp<+/-,32,32> 0.0 ("fixed-point type")
                  n234 = Unbundle(w663) -> ("First Correlation"=w662:i32, "Latest Correlation"=w654:i32)
                  n235 = Unbundle(w664) -> ("First Detector Count"=w660:i32)  [unwired: 3 out]
                  n236 = Scale By Power Of 2(n=i16 0, x=w661) -> (x*2^n=w652:fxp<+,32,0>)
                  n237 = Increment(x=w652) -> (x+1=w650:fxp<+,33,1>)
                  n238 = To Fixed-Point(fixed-point type=w653, number=w660) -> (fixed-point=w659:fxp<+/-,32,32>)
                  n239 = Bundle(cluster=w664, "First Detector Count"=w660, "Detector Gap Count"=w657) -> (w665:T8)  [unwired: 2 in]
                  n240 = To Fixed-Point(fixed-point type=w653, number=w657) -> (fixed-point=w656:fxp<+/-,32,32>)
                  n241 = Multiply(x=w650, y=w659) -> (x*y=w658:fxp<+/-,64,33>)
                  n242 = Bundle(cluster=w663, "First Correlation"=w662, "Latest Correlation"=w654) -> (w666:T9)
                  n243 = Less?(x=w658, y=w656) -> (x < y?=w655:bool)
                }
              }
              n244 = Greater?(x=w625, y=w624) -> (0:w623:bool)
              n245 = Or(x=w617, y=w623) -> (x .or. y?=w619:bool)
              n246 = case shown="False" w619 {
                tunnel: w640 -> [w644 _]
                tunnel: [w643 _] -> w638
                tunnel: [_ u8 11 ("Det 3")] -> w620
                frame False {
                  n247 = Less Or Equal To 0?(x=w644) -> (x <= 0?=w642:bool)
                  n248 = case shown="True" w642 {
                    tunnel: [u8 12 ("Det 3") u8 11 ("Det 3")] -> w643
                    frame True {
                    }
                    frame False {
                    }
                  }
                }
                frame True {
                }
              }
            }
            frame 12 {
              # "Wait for the particle to get to the second detector."
              n249 = Increment(x=w674) -> (x+1=w671:T9)
              n250 = Unbundle By Name(w672) -> ("Detector Max Speed Count"=w670:i32)
              n251 = Unbundle By Name(w671) -> ()  [unwired: 1 out]
              n252 = Greater Or Equal?(y=w670) -> (x >= y?=w669:bool)  [unwired: 1 in]
              n253 = case shown="True" w669 {
                tunnel: [u8 13 ("State") u8 12 ("State")] -> w668
                frame True {
                }
                frame False {
                }
              }
            }
            frame 13 {
              (unwired) 0 ("Second Detector Final Count")
              # "Waits for a reverse correlation that's close to the first two correlations."
              n254 = Increment(x=w694) -> (x+1=w679:T9)
              n255 = Unbundle By Name(w686) -> ("First Detector Count"=w685:i32)
              n256 = Unbundle By Name(w693) -> ("Detector Min Speed Count"=w692:i32)
              n257 = Unbundle By Name(w679) -> ()  [unwired: 1 out]
              n258 = Greater Or Equal?(y=w692) -> (x >= y?=w683:bool)  [unwired: 1 in]
              n259 = case shown="False" w683 {
                tunnel: [_ w715] -> w687
                tunnel: [u8 13 _] -> w691
                tunnel: w690 -> [_ w714]
                tunnel: w682 -> [_ w711]
                tunnel: w685 -> [_ w702]
                tunnel: [_ w700] -> _
                frame True {
                }
                frame False {
                  w698 = fxp<+/-,32,32> 0.0 ("fixed-point type")
                  n260 = Scale By Power Of 2(n=i16 0, x=w714) -> (x*2^n=w697:fxp<+,32,0>)
                  n261 = Unbundle By Name(w711) -> ("Filter 1.Det 2"=w708:i32, "Filter 3.Det 2"=w710:i32, "Filter 4.Det 2"=w709:i32)
                  n262 = To Fixed-Point(fixed-point type=w698, number=w702) -> (fixed-point=w705:fxp<+/-,32,32>)
                  n263 = Subtract(x=fxp<+,1,1> 1.0, y=w697) -> (x-y=w712:fxp<+,33,1>)
                  n264 = Add(x=w710, y=w709) -> (x+y=w707:i32)
                  n265 = Multiply(x=w712, y=w705) -> (x*y=w706:fxp<+/-,64,32>)
                  n266 = Subtract(x=w708, y=w707) -> (x-y=w701:i32)
                  n267 = To Fixed-Point(fixed-point type=w698, number=w701) -> (fixed-point=w704:fxp<+/-,32,32>)
                  n268 = Greater?(x=w704, y=w706) -> (0:w699:bool)
                  n269 = case shown="True" w699 {
                    tunnel: [u8 14 u8 13] -> w715
                    frame True {
                    }
                    frame False {
                    }
                  }
                  n270 = Bundle(cluster=T9 {"First Correlation"=0, "Latest Correlation"=0} ("input cluster"), "First Correlation"=w702, "Latest Correlation"=w701) -> (w700:T9)
                }
              }
              n271 = Add(x=w689, y=w688) -> ()  [unwired: 1 out]
              n272 = Unbundle(w679) -> (w681:i32, w678:i32, w677)
              n273 = Bundle(cluster=w679, w681, w678, w677) -> (w680:T9)
            }
            frame 14 {
              # "Searches for a maximum correlation. If the maximum correlation happens\nafter the speed limit, this isn't the right filter, and we go back to the beginning.\nIf the maximum correlation is too big, we also go back to the beginning."
              n274 = Decrement(x=w742) -> (x-1=w741:i32)
              n275 = Unbundle By Name(w734) -> ("Filter 1.Det 2"=w725:i32, "Filter 3.Det 2"=w733:i32, "Filter 4.Det 2"=w732:i32)
              n276 = Unbundle By Name(w727) -> ("Gap Min Speed Count"=w726:i32)
              n277 = Unbundle By Name(w736) -> ("Detector Gap Count"=w729:i32)
              n278 = Add(x=w733, y=w732) -> (x+y=w724:i32)
              n279 = Subtract(x=w725, y=w724) -> (x-y=w735:i32)
              n280 = Increment(x=w740) -> (x+1=w728:T9)
              n281 = Add(x=w729) -> (x+y=w730:i32)  [unwired: 1 in]
              n282 = Greater?(x=w735, y=w730) -> (0:w738:bool)
              n283 = case shown="True" w738 {
                tunnel: [w749 w768] -> w731
                tunnel: w728 -> [w749 w765]
                tunnel: w735 -> [_ w760]
                tunnel: [w750 w767] -> w737
                tunnel: w736 -> [w750 w766]
                tunnel: [_ w756] -> _
                tunnel: w721 -> [_ w752]
                tunnel: [_ w758] -> w720
                frame False {
                }
                frame True {
                  (unwired) 0 ("Second Detector Final Count")
                  w755 = fxp<+/-,32,32> 0.0 ("fixed-point type")
                  n284 = Scale By Power Of 2(n=i16 0, x=w752) -> (x*2^n=w754:fxp<+,32,0>)
                  n285 = Unbundle(w765) -> (w764:i32, w757:i32, w756)
                  n286 = Unbundle(w766) -> ("First Detector Count"=w763:i32)  [unwired: 3 out]
                  n287 = Increment(x=w754) -> (x+1=w751:fxp<+,33,1>)
                  n288 = Bundle(cluster=w765, w764, w757, w756) -> (w768:T9)
                  n289 = To Fixed-Point(fixed-point type=w755, number=w763) -> (fixed-point=w762:fxp<+/-,32,32>)
                  n290 = Bundle(cluster=w766, "First Detector Count"=w763, "Detector Gap Count"=w760) -> (w767:T8)  [unwired: 2 in]
                  n291 = To Fixed-Point(fixed-point type=w755, number=w760) -> (fixed-point=w759:fxp<+/-,32,32>)
                  n292 = Multiply(x=w751, y=w762) -> (x*y=w761:fxp<+/-,64,33>)
                  n293 = Less?(x=w761, y=w759) -> (x < y?=w758:bool)
                }
              }
              n294 = Greater?(y=w726) -> (0:w718:bool)  [unwired: 1 in]
              n295 = And(x=w720, y=w718) -> (x .and. y?=w722:bool)
              n296 = case shown="False" w722 {
                tunnel: w741 -> [w745 _]
                tunnel: [w744 _] -> w739
                tunnel: [_ u8 14 ("Det 3")] -> w723
                frame False {
                  n297 = Less Or Equal To 0?(x=w745) -> (x <= 0?=w743:bool)
                  n298 = case shown="False" w743 {
                    tunnel: [u8 15 ("Det 3") u8 14 ("Det 3")] -> w744
                    frame True {
                    }
                    frame False {
                    }
                  }
                }
                frame True {
                }
              }
            }
            frame 15 {
              # "v = clockspeed * distance / speed count"
              # "1/2mv^2 = Vq\ntherefore\nm = 2Vq/v^2"
              n299 = Increment(x=w803) -> (x+1=w802:T9)
              n300 = Unbundle By Name(w804) -> ("High Velocity Limit"=w787:fxp<+,18,18>, "Low Velocity Limit"=w788:fxp<+,18,18>, "High Mass Limit"=w797:fxp<+/-,33,-36>, "Low Mass Limit"=w772:fxp<+/-,33,-36>, "High Voltage"=w792:fxp<+,32,22>)
              n301 = Unbundle By Name(w802) -> ()  [unwired: 2 out]
              n302 = Multiply(x=w792, y=w776) -> (x*y=w798:fxp<+,64,-19>)
              n303 = Subtract() -> (x-y=w775:dbl)  [unwired: 2 in]
              n304 = To Fixed-Point(fixed-point type=fxp<+/-,32,32> 0.0, number=w775) -> (fixed-point=w786:fxp<+/-,32,32>)
              n305 = To Fixed-Point(fixed-point type=fxp<+,16,16> 0.0, number=w775) -> (fixed-point=w777:fxp<+,16,16>)
              n306 = Divide(x=w774, y=w775) -> (x/y=w773:dbl)
              n307 = Square(x=w777) -> (x^2=w778:fxp<+,32,32>)
              n308 = Multiply(x=w787, y=w786) -> (x*y=w785:fxp<+/-,50,50>)
              n309 = Multiply(x=w786, y=w788) -> (x*y=w784:fxp<+/-,50,50>)
              n310 = Multiply(x=w800, y=w778) -> (x*y=w799:fxp<+/-,64,-10>)
              n311 = To Fixed-Point(fixed-point type=fxp<+/-,32,-12> 0.0, number=w799) -> (fixed-point=w770:fxp<+/-,32,-12>)
              n312 = Greater Or Equal?(x=w785, y=w774) -> (x >= y?=w796:bool)
              n313 = Less Or Equal?(x=w784, y=w774) -> (x <= y?=w795:bool)
              n314 = Multiply(x=w798, y=w770) -> (x*y=w779:fxp<+/-,64,-31>)
              n315 = Scale By Power Of 2(n=i16 1, x=w779) -> (x*2^n=w771:fxp<+/-,64,-31>)
              n316 = Less Or Equal?(x=w771, y=w797) -> (x <= y?=w794:bool)
              n317 = Greater Or Equal?(x=w771, y=w772) -> (x >= y?=w793:bool)
              n318 = Compound Arithmetic op=AND(w796, w795, w794, w793, w783) -> (w782:bool)
              n319 = case shown="True" w782 {
                tunnel: [u8 16 ("Det 3") _] -> w790
                tunnel: [_ u8 15 ("Det 3")] -> w789
                frame True {
                }
                frame False {
                }
              }
            }
            frame 16 {
              n320 = Increment(x=w821) -> (x+1=w820:T9)
              n321 = Unbundle By Name(w820) -> ()  [unwired: 2 out]
              n322 = Subtract() -> (x-y=w817:dbl)  [unwired: 2 in]
              n323 = To Fixed-Point(fixed-point type=fxp<+/-,32,32> 0.0, number=w817) -> (fixed-point=w819:fxp<+/-,32,32>)
              n324 = Multiply(x=w819, y=w818) -> (x*y=w816:T12)
              n325 = To Long Integer(number=w816) -> (32bit integer=w815:T13)
              n326 = Subtract(x=w815, y=w814) -> (x-y=w813:T13)
              n327 = Subtract(x=w813) -> (x-y=w811:T13)  [unwired: 1 in]
              n328 = Unbundle By Name(w811) -> ("Distance to DCS 1"=w809:i32)
              n329 = Add(x=w809, y=w810) -> (x+y=w808:i32)
            }
            frame 17 {
              n330 = Decrement(x=w826) -> (x-1=w825:T13)
              n331 = Unbundle By Name(w825) -> ("Distance to PSU"=w824:i32)
              n332 = Less Or Equal To 0?(x=w824) -> (x <= 0?=w822:bool)
              n333 = case shown="True" w822 {
                tunnel: [u8 18 ("Det 3") u8 17 ("Det 3")] -> w823
                frame True {
                }
                frame False {
                }
              }
            }
            frame 18 {
              n334 = Decrement(x=w834) -> (x-1=w833:T13)
              n335 = Unbundle By Name(w833) -> ("Distance to end of PSU"=w832:i32)
              n336 = Less Or Equal To 0?(x=w832) -> (x <= 0?=w830:bool)
              n337 = case shown="True" w830 {
                tunnel: [u8 19 ("Det 3") u8 18 ("Det 3")] -> w831
                frame True {
                }
                frame False {
                }
              }
            }
            frame 19 {
              n338 = Decrement(x=w841) -> (x-1=w840:T13)
              n339 = Unbundle By Name(w840) -> ("Distance to DCS 2"=w839:i32)
              n340 = Less Or Equal To 0?(x=w839) -> (x <= 0?=w837:bool)
              n341 = case shown="True" w837 {
                tunnel: [u8 20 ("Det 3") u8 19 ("Det 3")] -> w838
                frame True {
                }
                frame False {
                }
              }
            }
            frame 20 {
              n342 = Decrement(x=w850) -> (x-1=w849:T13)
              n343 = Unbundle By Name(w849) -> ("Distance to DCS 2"=w848:i32)
              n344 = Add(x=w848, y=w847) -> (x+y=w846:i32)
              n345 = Less Or Equal To 0?(x=w846) -> (x <= 0?=w845:bool)
              n346 = case shown="True" w845 {
                tunnel: [u8 20 ("Det 3") w855] -> w852
                tunnel: w844 -> [_ w854]
                frame False {
                }
                frame True {
                  n347 = case shown="True" w854 {
                    tunnel: [_ u8 21 ("Det 3")] -> w855
                    frame False {
                    }
                    frame True {
                    }
                  }
                }
              }
            }
            frame 21 {
              n348 = Decrement(x=w861) -> (x-1=w860:T13)
              n349 = Unbundle By Name(w860) -> ("Distance to front of LEIL Chamber"=w859:i32)
              n350 = Less Or Equal To 0?(x=w859) -> (x <= 0?=w857:bool)
              n351 = case shown="True" w857 {
                tunnel: [u8 22 ("Det 3") u8 21 ("Det 3")] -> w858
                frame True {
                }
                frame False {
                }
              }
            }
            frame 22 {
              n352 = Decrement(x=w870) -> (x-1=w869:T13)
              n353 = Unbundle By Name(w869) -> ("Distance to front of LEIL Chamber"=w868:i32)
              n354 = Add(x=w868, y=w867) -> (x+y=w866:i32)
              n355 = Less Or Equal To 0?(x=w866) -> (x <= 0?=w865:bool)
              n356 = case shown="False" w865 {
                tunnel: [u8 22 ("Det 3") _] -> w871
                frame False {
                }
                frame True {
                }
              }
            }
          }
        }
      }
      n357 = disable-structure shown="Disabled" {
        disable-tunnel: w249 -> [w898 w906]
        disable-tunnel: [w894 w905] -> w245
        disable-tunnel: [w896 _] -> w244
        disable-tunnel: w243 -> [w897 _]
        frame Disabled {
          n358 = case shown="1, Default" w898 {
            selector: w898 -> [_ w904]
            tunnel: [w901 w902] -> w895
            tunnel: w897 -> [w901 w903]
            frame 0 {
            }
            frame 1, Default {
              n359 = Max & Min(x=w904, y=w903) -> (min(x,y)=w902:i32)  [unwired: 1 out]
            }
          }
          n360 = Less Than 0?(x=w895) -> (x < 0?=w894:bool)
          n361 = case shown="False" w894 {
            tunnel: w895 -> [w900 _]
            tunnel: [w899 _] -> w896
            frame False {
              n362 = Decrement(x=w900) -> (x-1=w899:i32)
            }
            frame True {
            }
          }
        }
        frame Enabled {
          n363 = Not Equal To 0?(x=w906) -> (x != 0?=w905:bool)
        }
      }
      n364 = case shown="False" w223 {
        tunnel: w238 -> [w878 w885]
        tunnel: w237 -> [w879 w886]
        tunnel: w236 -> [w881 w887]
        tunnel: [w876 w884] -> w224
        tunnel: w230 -> [w883 _]
        frame False {
          n365 = Unbundle(w883) -> (w882:dbl, w880:fxp<+/-,64,-31>, "High Charge Limit"=w877:fxp<+,32,-41>)
          n366 = To Fixed-Point(fixed-point type=w879, number=w880) -> (fixed-point=w874:fxp<+/-,64,-31>)
          n367 = To Fixed-Point(fixed-point type=w878, number=w877) -> (fixed-point=w873:fxp<+,32,-41>)
          n368 = To Fixed-Point(fixed-point type=w881, number=w882) -> (fixed-point=w875:fxp<+,64,32>)
          n369 = Bundle(w875, w874, "High Charge Limit"=w873) -> (w876:T14)  [unwired: 1 in]
        }
        frame True {
          n370 = Bundle(w887, w886, "High Charge Limit"=w885) -> (w884:T15)  [unwired: 1 in]
        }
      }
      n371 = case shown="False" w245 {
        tunnel: w248 -> [_ w893]
        tunnel: [w888 w893] -> w247
        tunnel: w246 -> [w889 _]
        frame False {
          n372 = case shown="1, Default" w889 {
            selector: w889 -> [w890 w892]
            tunnel: [w890 w891] -> w888
            frame 0 {
            }
            frame 1, Default {
              n373 = Decrement(x=w892) -> (x-1=w891:u16)
            }
          }
        }
        frame True {
        }
      }
    }
    n374 = case shown="True" "Calibrate" {
      tunnel: w164 -> [w208 _]
      tunnel: w129 -> [w210 w213]
      tunnel: [w210 w211] -> w179
      tunnel: w163 -> [_ w212]
      tunnel: [w209 _] -> w128
      tunnel: w117 -> [w207 _]
      frame False {
        n375 = Index Array(array=w208, index=w207) -> (element=w209:u8)
      }
      frame True {
        n376 = for {
          tunnel: w212 -> [w216] mode=indexing
          tunnel: w213 -> [w215] mode=indexing
          tunnel: [w214] -> w211 mode=indexing
          n377 = Max & Min(x=w215, y=w216) -> (max(x,y)=w214:i32)  [unwired: 1 out]
        }
      }
    }
    n378 = case shown="1, Default" w126 {
      tunnel: [_ w198] -> w125
      tunnel: w124 -> [_ w198]
      frame 0 {
      }
      frame 1, Default {
      }
    }
    n379 = Or Array Elements(Boolean array=w145) -> (logical OR=w139:bool)
    n380 = Not(x=w139) -> (.not. x?=w144:bool)
    n381 = Or Array Elements(Boolean array=w150) -> (logical OR=w136:bool)
    "Plates" <- w136
    n382 = Or Array Elements(Boolean array=w149) -> (logical OR=→"DCS 2":bool)
    n383 = Or Array Elements(Boolean array=w148) -> (logical OR=→"User Trigger":bool)
    n384 = Greater Than 0?(x=w173) -> (x > 0?=w160:bool[])
    n385 = And(x=w144, y=w142) -> (x .and. y?=w143:bool)
    n386 = Or Array Elements(Boolean array=w160) -> (logical OR=→"DCS 1":bool)
    n387 = local write "Armed"(w143) -> ()
  }
  "PSU Response" <- w29
  "Thresholds out" <- w39
  n388 = local read "Max Stop Point"() -> (w25:cluster{"Max Stop":u8, "Index":i32})
  n389 = Array Max & Min(array=w28) -> (max value=w27:u8, max index (indices)=w1:i32)  [unwired: 2 out]
  n390 = Bundle(cluster=w25, "Max Stop"=w27, "Index"=w1) -> (→"Max Stop Point":cluster{"Max Stop":u8, "Index":i32})
  n391 = To Single Precision Float(number=w18) -> (single precision float=w17:cluster{sgl, sgl, "High Charge Limit":sgl}[])
  n392 = for {
    tunnel: w17 -> [w908] mode=indexing
    tunnel: [w907] -> w15 mode=indexing
    n393 = Cluster To Array(cluster=w908) -> (array=w907:sgl[])
  }
  n394 = Transpose 2D Array(2D array=w15) -> (transposed array=w13:sgl[][])
  n395 = Index Array(array=w13) -> (element=w14:sgl[])  [unwired: 2 in]
  n396 = Not Equal To 0?(x=w14) -> (x != 0?=w16:bool[])
  n397 = Boolean To (0,1)(Boolean=w16) -> (0, 1=w21:i16[])
  n398 = Add Array Elements(numeric array=w21) -> (sum=w19:i16)
  n399 = for {
    N: w19 -> [_]
    tunnel: w13 -> [w912]
    tunnel: w16 -> [w914]
    shift-right: [w910] -> _
    shift-left: -1 ("index of element") -> [w915]
    tunnel: [w909] -> w12 mode=indexing
    n400 = Increment(x=w915) -> (x+1=w911:i32)
    n401 = Search 1D Array(1D array=w914, element=TRUE, start index (0)=w911) -> (index of element=w910:i32)
    n402 = Index Array(array=w912, index (col)=w910) -> (element=w909:sgl[])  [unwired: 1 in]
  }
  n403 = Transpose 2D Array(2D array=w12) -> (transposed array=w11:sgl[][])
  n404 = for {
    tunnel: w11 -> [w919] mode=indexing
    tunnel: [w916] -> w10 mode=indexing
    n405 = Add Array Elements(numeric array=w919) -> (sum=w918:sgl)
    n406 = Array Size(array=w919) -> (size(s)=w917:i32)
    n407 = Divide(x=w918, y=w917) -> (x/y=w916:sgl)
  }
  "V-M-C Estimate" <- w10
